vi "SaveData.vi"   [LabVIEW 2011, in "OfflineTracker.lvlib"]
uses:
  OfflineTracker.lvlib
  <vilib>/Utility/file.llb/Write To Spreadsheet File (DBL).vi
types:
  T1 = enum16{"init", "get", "set single frame", "set all"}
  T2 = typedef "IMAQ Image.ctl" = refnum<image>
  T3 = cluster{"front panel settings":cluster{"files":cluster{"LUT path":path, "Trace path":path, " folders #":i32, "base path":path, "use trace":bool, "use base":bool, "LUT tmp":i32, "Trace tmp":i32, "active path":path}, "Tracking":cluster{"RminZ (pix)":i32, "Rmax (pix)":i32, "angular pixel \ncoverage factor":dbl, "radial pixel \ncoverage factor":dbl}, "Frames":cluster{"Start frame":i32, "number of frames":u32, "display frame ":i32, "track every nd frame ":i32, "Track all frames":bool, "active frame":i32}, "Calibs":cluster{"Zlut number of steps":i32, "pix/um":dbl, "Z correction factor":dbl, "Zlut step size (um)":dbl, "ROI(pix)":i32}, "Beads":cluster{"number of ref beads":i32, "overlay":bool}, "Misc":cluster{"save images to new location":bool, "destination":path}}, "data":cluster{"Image":T2, "image size":i32[], "Bead Array":i32[][], "overlay image":T2, "# beads":i32, "Job list":string[][], "job running":bool, "job #":i32, "folders to go":i32}}
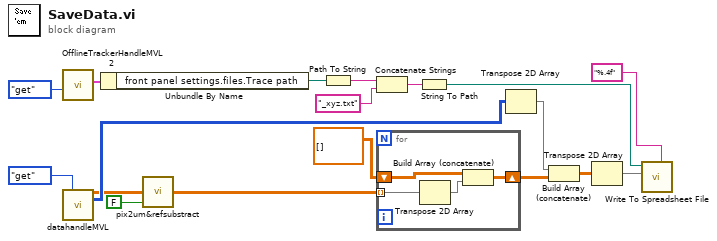
[diagram p0: block diagram]
diagram:
  n1 = call "OfflineTrackerHandleMVL2.vi"("action"=enum16{"get", "set"}."get") -> ("out"=w8:T3)  [unwired: 5 in, 1 out]
  n2 = call "datahandleMVL.vi"("action"=T1."get") -> ("XYZ out"=w11:dbl[][][], "time out"=w17:i32[][])  [unwired: 9 in, 4 out]
  n3 = Unbundle By Name(w8) -> ("front panel settings.files.Trace path"=w7:path)
  n4 = call "pix2um&refsubstract.vi"("ref substract"=FALSE, "XYZ in"=w11) -> ("xyz um out"=w12:dbl[][][])  [unwired: 3 out]
  n5 = Path To String(path=w7) -> (string=w3:string)
  n6 = Concatenate Strings(w3, "_xyz.txt" ("string")) -> (w2:string)
  n7 = for {
    tunnel: w12 -> [w20] mode=indexing
    shift-right: [w22] -> w15
    shift-left: dbl[][] [] ("xyz um out") -> [w21]
    n8 = Transpose 2D Array(2D array=w20) -> (transposed array=w19:dbl[][])
    n9 = Build Array (concatenate)(w21, w19) -> (w22:dbl[][])
  }
  n10 = String To Path(string=w2) -> (path=w1:path)
  n11 = Transpose 2D Array(2D array=w17) -> (transposed array=w18:i32[][])
  n12 = Build Array (concatenate)(w18, w15) -> (w16:dbl[][])
  n13 = Transpose 2D Array(2D array=w16) -> (transposed array=w4:dbl[][])
  n14 = call-poly <vilib>:"Write To Spreadsheet File.vi"("format (%.3f)"="%.4f", "2D data"=w4, "file path (dialog if empty)"=w1) -> ()  [unwired: 3 in, 3 out]
